vi "Plugin Configuration.Get Timing.vi"(11 "Plugin Configuration in":refnum<class "Plugin Configuration.lvclass">) -> (2 "cycle timing":T1={"priority"=0, "decimation"=1, "offset"=0}, 3 "Plugin Configuration out":refnum<class "Plugin Configuration.lvclass">)   [LabVIEW 2017, in "DSF Core.lvlib" / "Plugin Configuration.lvclass"]
uses:
  Plugin Configuration.lvclass
  DSF Configuration API/Public/Controls/DSF Timing Info.ctl
  Plugin Configuration.lvclass/Plugin Configuration.ctl
  DSF Core.lvlib
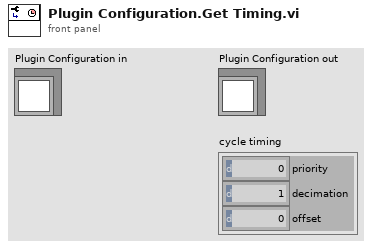
[diagram p1: front panel]
types:
  T1 = typedef "DSF Core.lvlib/DSF Timing Info.ctl" = cluster{"priority":u64, "decimation":u64, "offset":u64}
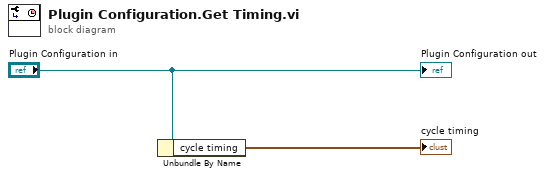
[diagram p0: block diagram]
diagram:
  n1 = Unbundle By Name("Plugin Configuration in") -> ("cycle timing"=→"cycle timing":T1)
  "Plugin Configuration out" <- "Plugin Configuration in"
